vi "Evaluate Checksum.vi"(5 "Subroutine in":refnum<class "Subroutine.lvclass">, 6 "Path Builder":refnum<class "IPath Builder.lvclass">, 7 "Linked List ID":string, 8 "error in (no error)":errorcluster, 11 "Linked List Ref":refnum<data-value>) -> (0 "error out":errorcluster, 1 "Checksum Match":bool, 2 "Path":path, 3 "Linked List Ref out":refnum<data-value>)   [LabVIEW 2020, in "Test Executive.lvlib" / "Subroutine.lvclass"]
uses:
  <vilib>/gpm_packages/@cs/test-executive/Source/Test Executive/Subroutine/Subroutine.lvclass
  <vilib>/gpm_packages/@cs/linked-list/Source/Linked List/ILinkedList/ILinked List.lvclass
  <vilib>/gpm_packages/@cs/test-executive/Source/Path Builder/IPath Builder/IPath Builder.lvclass
  <vilib>/gpm_packages/@cs/linked-list/Source/Linked List/Linked List Ref/Linked List Ref.lvclass
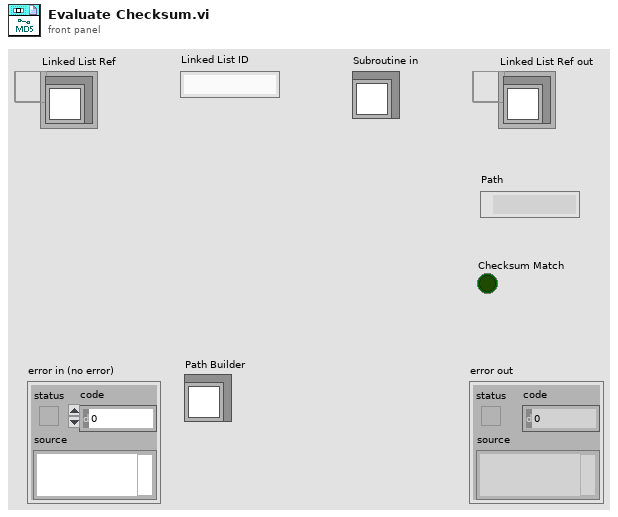
[diagram p1: front panel]
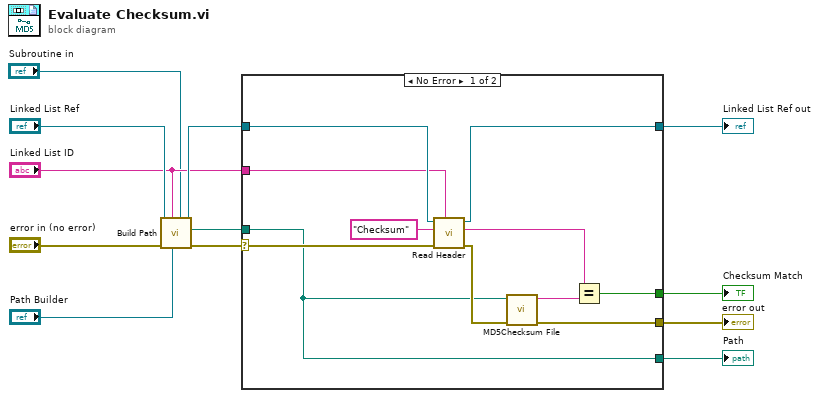
[diagram p0: block diagram]
diagram:
  n1 = call-dynamic "Build Path.vi"("Subroutine in"="Subroutine in", "Path Builder"="Path Builder", "Linked List ID"="Linked List ID", "error in (no error)"="error in (no error)", "Linked List Ref"="Linked List Ref") -> ("error out"=w5:errorcluster, "Path"=w3:path, "Linked List Ref out"=w8:refnum<data-value>)  [unwired: 4 in]
  n2 = case shown="No Error" w5 {
    selector: w5 -> [w14 w24]
    tunnel: [w20 _] -> w12
    tunnel: [w19 w25] -> w11
    tunnel: [w17 w24] -> w10
    tunnel: w8 -> [w16 w25]
    tunnel: "Linked List ID" -> [w15 _]
    tunnel: w3 -> [w13 _]
    tunnel: [w13 _] -> w2
    frame No Error {
      n3 = call <vilib>:"Read Header.vi"("Linked List ID"=w15, "error in (no error)"=w14, "Header Name"="Checksum", "Linked List Ref"=w16) -> ("error out"=w18:errorcluster, "Header Value"=w21:string, "Linked List Ref out"=w19:refnum<data-value>)  [unwired: 4 in, 1 out]
      n4 = call <vilib>:"MD5Checksum File.vi"("error in (no error)"=w18, "Path"=w13) -> ("error out"=w17:errorcluster, "MD5 message-digest"=w22:string)  [unwired: 8 in]
      n5 = Equal?(x=w21, y=w22) -> (x = y?=w20:bool)
    }
    frame Error {
    }
  }
  "Linked List Ref out" <- w11
  "error out" <- w10
  "Checksum Match" <- w12
  "Path" <- w2
